vi "Read Attributes.vi"(11 "New Data Msg":refnum<class "New Data Msg.lvclass">) -> (2 "Payload":cluster{"String Data":string})   [LabVIEW 2015, in "Nested Actor.lvlib" / "New Data Msg.lvclass"]
uses:
  New Data Msg.lvclass
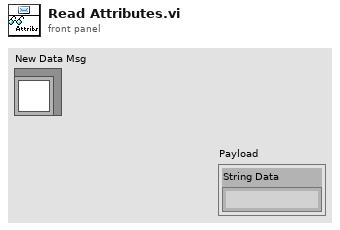
[diagram p1: front panel]
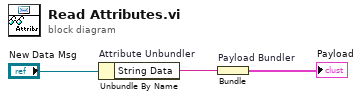
[diagram p0: block diagram]
diagram:
  n1 = Unbundle By Name "Attribute Unbundler"("New Data Msg") -> ("String Data"=w1:string)
  n2 = Bundle "Payload Bundler"("String Data"=w1) -> (→"Payload":cluster{"String Data":string})  [unwired: 1 in]
